vi "time-str-to-time-dbl-RA.vi"(1 "Chaîne":string) -> (0 "TCS_coords":dbl format="%.5f")   [LabVIEW 2019]
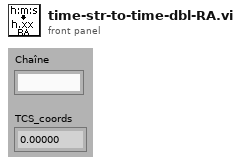
[diagram p1: front panel]
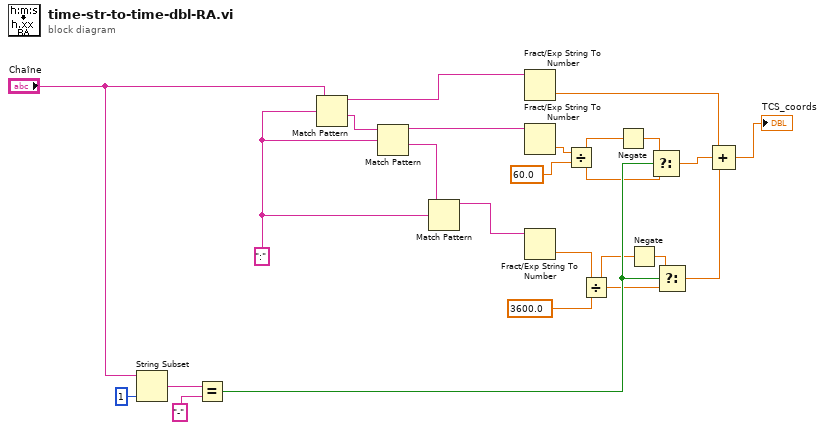
[diagram p0: block diagram]
diagram:
  w13 = ":"
  n1 = String Subset(string="Chaîne", length (rest)=1 ("length (rest)")) -> (substring=w10:string)  [unwired: 1 in]
  n2 = Equal?(x=w10, y="-") -> (x = y?=w8:bool)
  n3 = Match Pattern(string="Chaîne", regular expression=w13) -> (before substring=w20:string, after substring=w22:string)  [unwired: 1 in, 2 out]
  n4 = Match Pattern(string=w22, regular expression=w13) -> (before substring=w19:string, after substring=w21:string)  [unwired: 1 in, 2 out]
  n5 = Match Pattern(string=w21, regular expression=w13) -> (before substring=w18:string)  [unwired: 1 in, 3 out]
  n6 = Fract/Exp String To Number(string=w20) -> (number=w1:dbl)  [unwired: 3 in, 1 out]
  n7 = Fract/Exp String To Number(string=w19) -> (number=w17:dbl)  [unwired: 3 in, 1 out]
  n8 = Fract/Exp String To Number(string=w18) -> (number=w14:dbl)  [unwired: 3 in, 1 out]
  n9 = Divide(x=w17, y=60.0) -> (x/y=w5:dbl)
  n10 = Divide(x=w14, y=3600.0) -> (x/y=w6:dbl)
  n11 = Negate(x=w5) -> (-x=w4:dbl)
  n12 = Negate(x=w6) -> (-x=w7:dbl)
  n13 = Select(t=w4, s=w8, f=w5) -> (s? t:f=w3:dbl)
  n14 = Select(t=w7, s=w8, f=w6) -> (s? t:f=w2:dbl)
  n15 = Compound Arithmetic op=ADD(w1, w3, w2) -> (→"TCS_coords":dbl)
